vi "prefixTreeDelimiter.set.vi"(8 "error in (no error)":errorcluster, 10 "prefixTreeDelimiter":string, 11 "channelConfig in":refnum<class "channelConfig.lvclass">) -> (0 "error out":errorcluster, 3 "channelConfig out":refnum<class "channelConfig.lvclass">)   [LabVIEW 2020, in "nominal types.lvlib" / "channelConfig.lvclass"]
uses:
  channelConfig.lvclass
  channelConfig.lvclass/channelConfig.ctl
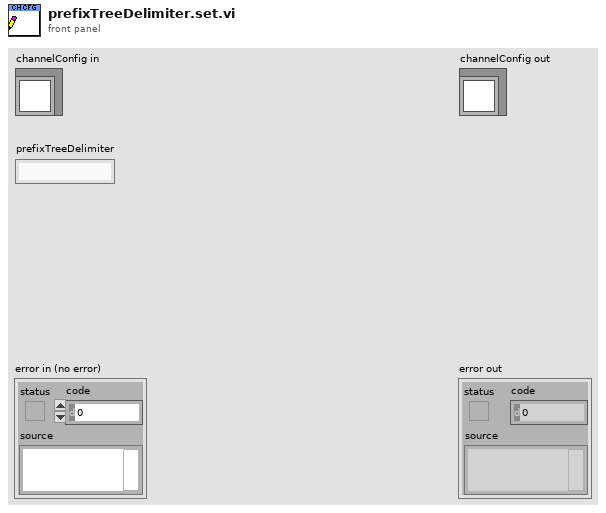
[diagram p1: front panel]
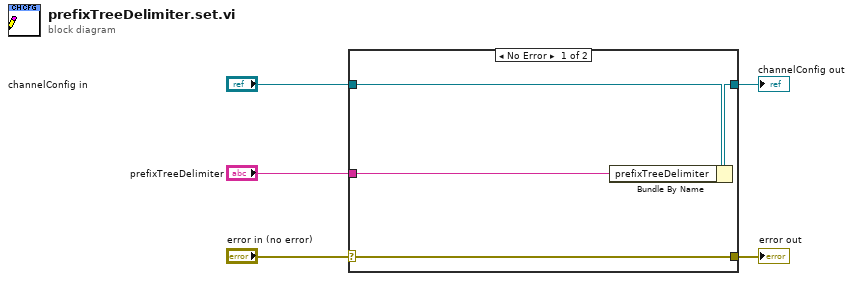
[diagram p0: block diagram]
diagram:
  n1 = case shown="No Error" "error in (no error)" {
    selector: "error in (no error)" -> [w9 w10]
    tunnel: [w9 w10] -> w4
    tunnel: [w7 w11] -> w2
    tunnel: "channelConfig in" -> [w8 w11]
    tunnel: "prefixTreeDelimiter" -> [w6 _]
    frame No Error {
      n2 = Bundle By Name(cluster=w8, "prefixTreeDelimiter"=w6) -> (w7:refnum<class "channelConfig.lvclass">)
    }
    frame Error {
    }
  }
  "error out" <- w4
  "channelConfig out" <- w2
